vi "Listener.vi"(10 "Stop":bool=TRUE, 11 "BT Queue":refnum<queue>) -> ()   [LabVIEW 2013, in "main.lvlib"]
uses:
  main.lvlib
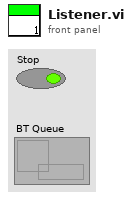
[diagram p1: front panel]
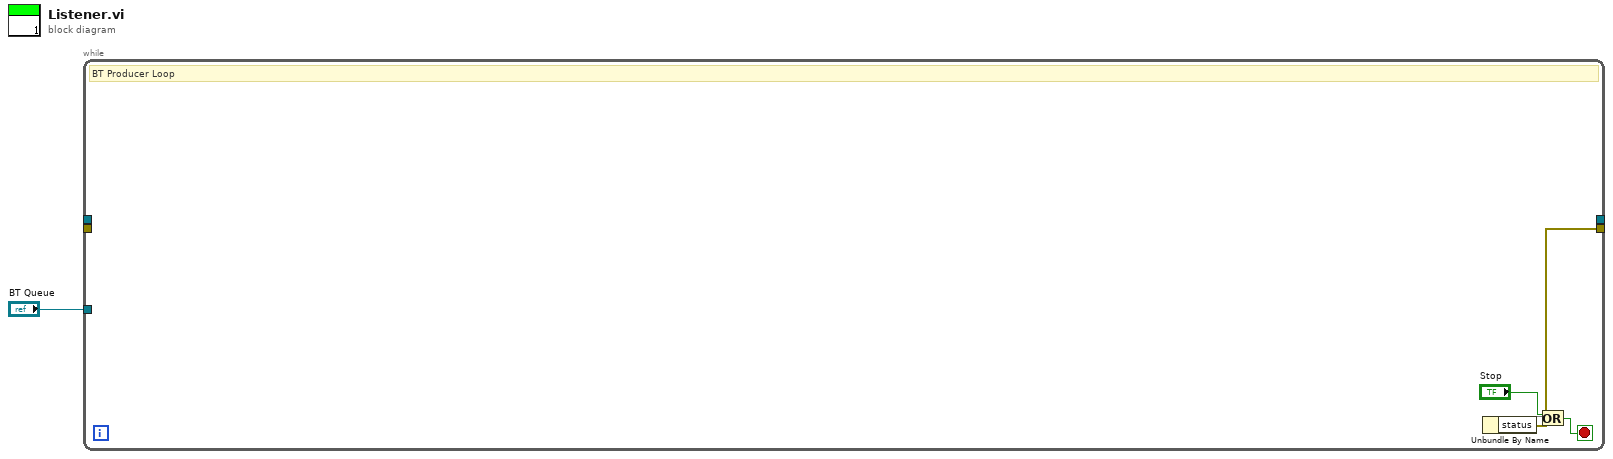
[diagram p0: block diagram]
diagram:
  n1 = while {
    tunnel: _ -> [w11]
    tunnel: [w8] -> _
    tunnel: [w10] -> w3
    tunnel: [w9] -> w2
    tunnel: "BT Queue" -> [w4]
    stop <- w5 stop-if-true
    # "BT Producer Loop"
    n2 = Unbundle By Name() -> (w8:errorcluster, "status"=w7)
    n3 = Or(x="Stop", y=w7) -> (x .or. y?=w5:bool)
  }
